vi "Idle_APCSwitchSetOutletName.vi"(0 "IP Address":string="192.168.0.130", 5 "Write Community String":string="private", 7 "timeout ms (750)":i32=750, 9 "Name":string="SampleName", 11 "ErrorIn":errorcluster, 12 "Outlet":u8=1 min=1 max=8 step=1) -> (15 "ErrorOut":errorcluster)   [LabVIEW 2012]
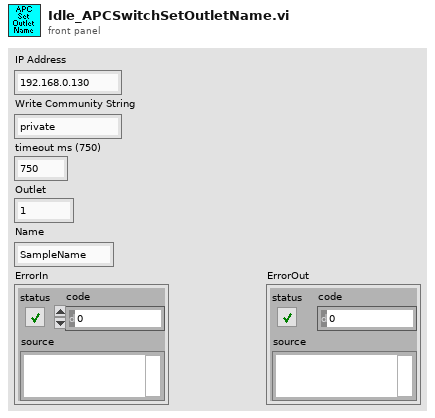
[diagram p1: front panel]
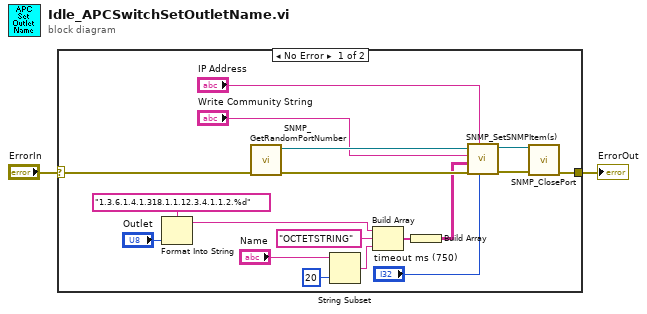
[diagram p0: block diagram]
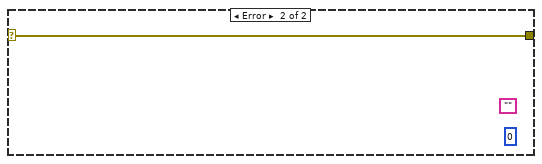
[diagram p2: hidden frame]
diagram:
  n1 = case shown="No Error" "ErrorIn" {
    selector: "ErrorIn" -> [w3 w21]
    tunnel: [w16 w21] -> w1
    frame No Error {
      n2 = Format Into String(format string="1.3.6.1.4.1.318.1.1.12.3.4.1.1.2.%d", "Outlet") -> (resulting string=w11:string)  [unwired: 2 in, 1 out]
      n3 = call "SNMP_GetRandomPortNumber.vi"("error in (no error)"=w3) -> ("error out"=w18:errorcluster, "connection ID"=w20:refnum<k16>)  [unwired: 9 out]
      n4 = String Subset(string="Name", length (rest)=20 ("length (rest)")) -> (substring=w5:string)  [unwired: 1 out]
      n5 = Build Array(w11, "OCTETSTRING", w5) -> (w10:string[])
      n6 = Build Array(w10) -> (w9:string[][])
      n7 = call "SNMP_SetSNMPItem(s).vi"("timeout ms (25000)"="timeout ms (750)", "IP Address of SNMP Device"="IP Address", "error in (no error)"=w18, "OID/TYPE/VALUE ARRAY"=w9, "Community Name"="Write Community String", "connection ID in"=w20) -> ("error out"=w17:errorcluster, "connection ID out"=w19:refnum<k16>)  [unwired: 4 out]
      n8 = call "SNMP_ClosePort.vi"("error in (no error)"=w17, "connection ID"=w19) -> ("error out"=w16:errorcluster)  [unwired: 9 out]
    }
    frame Error {
      (unwired) u8 0 ("error-status")
      (unwired) ""
    }
  }
  "ErrorOut" <- w1
